vi "ReadAPD_noise.vi"() -> ()   [LabVIEW 2019]
uses:
  <vilib>/DAQmx/read.llb/DAQmx Read (Analog Wfm 1Chan NSamp Duration).vi
  <vilib>/Analysis/5stat.llb/RMS (DBL).vi
  <vilib>/DAQmx/create/channels.llb/DAQmx Create Channel (AI-Voltage-Basic).vi
  <vilib>/DAQmx/miscellaneous.llb/DAQmx Fill In Error Info.vi
  <resource>/objmgr/daqmx.rc
  <vilib>/Analysis/NI_AALPro.lvlib
panel:
  out "rms value":dbl=0.0002525193524182887 format="%.3p"
  in  "Lockin Sensitivity":dbl=0.0001 format="%#_3p"
  out "APD Signal":waveform(dbl)(graph)={"t0"=timestamp(3741008050.867453 s since 1904-01-01), "dt"=0.0009999999888823368, "Y"=array[5000 elements], "attributes"=variant("NI_ChannelName"=variant(string "Dev1/ai0"), "NI_UnitDescription"=variant(string "Volts"))}
  in  "Sampling Clock":dbl=1000.0 format="%#_3p"
  in  "Input Channel":tag="Dev1/ai0"
  # "(10 for default)"
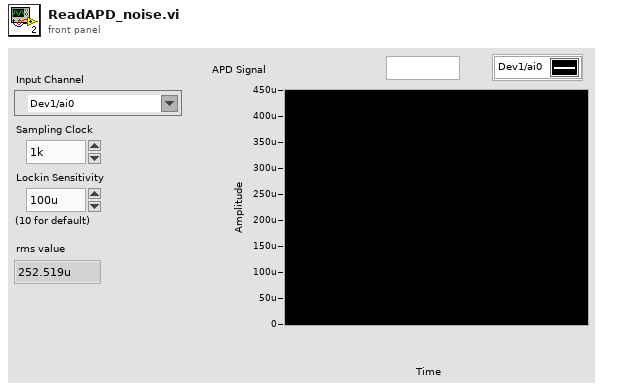
[diagram p1: front panel]
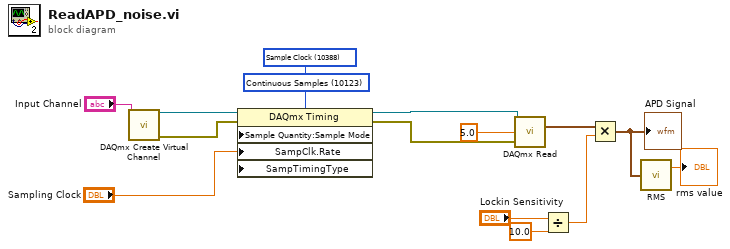
[diagram p0: block diagram]
diagram:
  w9 = 10388 items=["Sample Clock"=10388, "Burst Handshake"=12548, "Handshake"=10389, "Implicit"=10451, "On Demand"=10390, "Change Detection"=12504, "Pipelined Sample Clock"=14668] ("SampTimingType")
  w10 = 10123 items=["Finite Samples"=10178, "Continuous Samples"=10123, "Hardware Timed Single Point"=12522] ("SampQuant.SampMode")
  n1 = call-poly <vilib>:"DAQmx Create Virtual Channel.vi"("physical channels"="Input Channel") -> ("task out"=w14:refnum<k21>, "error out"=w12:errorcluster)  [unwired: 13 in]
  n2 = property class="DAQmx Timing"(reference=w14, error in=w12, "Sample Quantity:Sample Mode"=w10, "SampClk.Rate"="Sampling Clock", "SampTimingType"=w9) -> (reference out=w13:refnum<k21>, error out=w11:errorcluster)
  n3 = call-poly <vilib>:"DAQmx Read.vi"("task/channels in"=w13, "duration"=5.0, "error in"=w11) -> ("data"=w5:waveform(dbl))  [unwired: 10 in, 2 out]
  n4 = Divide(x="Lockin Sensitivity", y=10.0) -> (x/y=w4:dbl)
  n5 = Multiply(x=w5, y=w4) -> (x*y=w3:waveform(dbl))
  "APD Signal" <- w3
  n6 = call-poly <vilib>:"RMS.vi"("X"=w3) -> ("rms value"=→"rms value":dbl)  [unwired: 1 out]
